vi "Set default values.vi"(8 "error in (no error)":errorcluster, 11 "device data model in":refnum<class "WebSocket Data Model.lvclass">) -> (0 "error out":errorcluster, 3 "device data model out":refnum<class "WebSocket Data Model.lvclass">)   [LabVIEW 2021, in "WebSockets.lvlib" / "WebSocket Data Model.lvclass"]
doc: "This VI ensures that the data model has at least 65,535 values of every type. This is required for certain modbus function codes."
uses:
  WebSocket Data Model.lvclass
  WebSocket Data Model.lvclass/WebSocket Data Model.ctl
  Type Definitions/Data Model.ctl
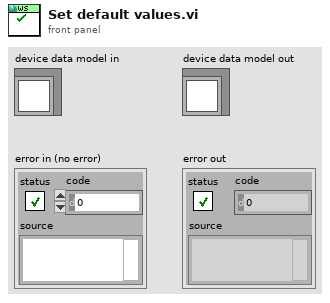
[diagram p1: front panel]
types:
  T1 = typedef "WebSockets.lvlib/WebSocket Data Model.lvclass/Data Model.ctl" = cluster{"UTC":u64, "Receive Binary Data":u8[], "Receive Text Data":string, "Send Binary Data":u8[], "Send Text Data":string, "ES":u8}
  T2 = typedef "Device Data Model.lvclass/N channel.ctl" = cluster{"N DI channel":i32, "N DO channel":i32, "N AI channel":i32, "N AO channel":i32}
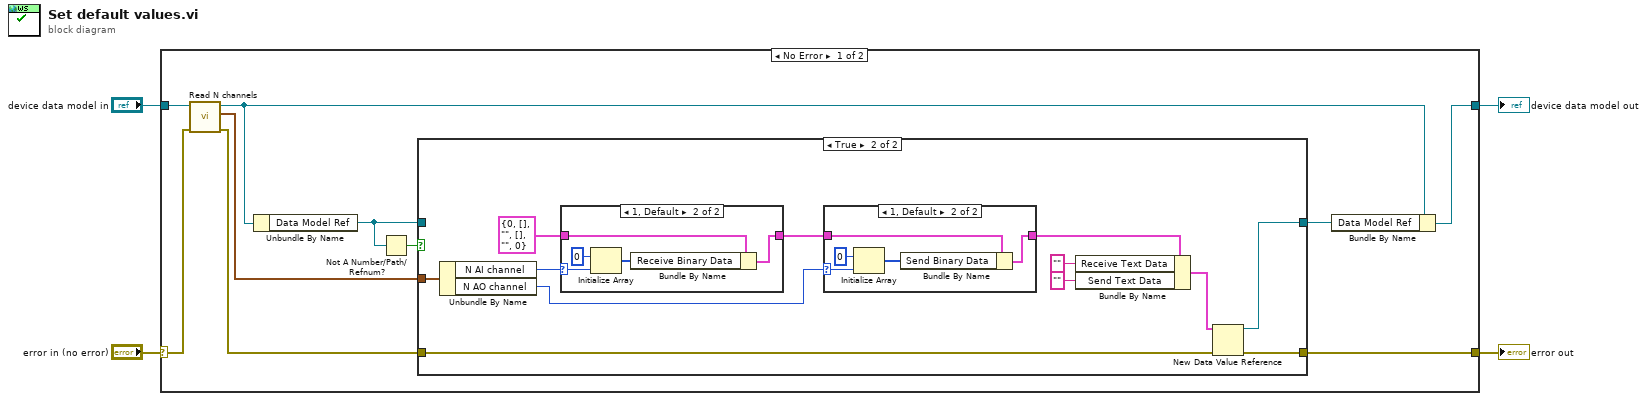
[diagram p0: block diagram]
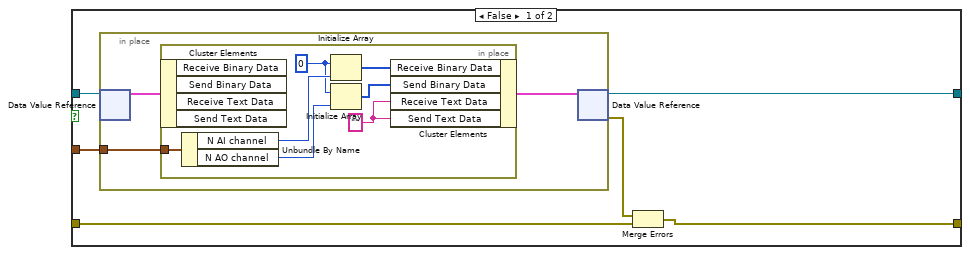
[diagram p2: hidden frame]
diagram:
  n1 = case shown="No Error" "error in (no error)" {
    selector: "error in (no error)" -> [w7 w56]
    tunnel: "device data model in" -> [w9 w55]
    tunnel: [w14 w55] -> w3
    tunnel: [w10 w56] -> w2
    frame No Error {
      n2 = call-dynamic "Read N channels.vi"("error in (no error)"=w7, "device data model in"=w9) -> ("error out"=w6:errorcluster, "N channel"=w5:T2, "device data model out"=w8:refnum<class "WebSocket Data Model.lvclass">)  [unwired: 7 in]
      n3 = Unbundle By Name(w8) -> ("Data Model Ref"=w12:refnum<data-value>)
      n4 = Not A Number/Path/Refnum?(number/path/refnum=w12) -> (NaN/Path/Refnum?=w11:bool)
      n5 = case shown="True" w11 {
        tunnel: w6 -> [w15 w42]
        tunnel: w12 -> [w20 _]
        tunnel: [w19 w40] -> w13
        tunnel: [w18 w41] -> w10
        tunnel: w5 -> [w16 w32]
        frame False {
          n6 = in-place {
            in-place-border: w16 -> [w22]
            n7 = in-place-dvr #1(w20) -> (w23:T1)  [unwired: 1 out]
            n8 = in-place {
              in-place-border: w22 -> [w30]
              w24 = "" ("Text Data")
              w26 = u8 0 ("Boolean")
              n9 = in-place-cluster #2(w23) -> ()  [unwired: 4 out]
              n10 = Unbundle By Name(w30) -> ("N AI channel"=w29:i32, "N AO channel"=w27:i32)
              n11 = Initialize Array(w26, w29) -> (w28:u8[])
              n12 = Initialize Array(w26, w27) -> (w25:u8[])
              n13 = in-place-cluster #2("Receive Binary Data"=w28, "Send Binary Data"=w25, "Receive Text Data"=w24, "Send Text Data"=w24) -> (w21:T1)
            }
            n14 = in-place-dvr #1(w21) -> (w19:refnum<data-value>, w17:errorcluster)
          }
          n15 = Merge Errors(w17, w15) -> (w18:errorcluster)
        }
        frame True {
          n16 = Unbundle By Name(w32) -> ("N AI channel"=w38:i32, "N AO channel"=w33:i32)
          n17 = case shown="1, Default" w38 {
            selector: w38 -> [_ w50]
            tunnel: T1 {"UTC"=0, "Receive Binary Data"=[], "Receive Text Data"="", "Send Binary Data"=[], "Send Text Data"="", "ES"=0} ("Data Model") -> [w49 w53]
            tunnel: [w49 w51] -> w35
            frame 0 {
            }
            frame 1, Default {
              n18 = Initialize Array(u8 0 ("Boolean"), w50) -> (w52:u8[])
              n19 = Bundle By Name(cluster=w53, "Receive Binary Data"=w52) -> (w51:T1)
            }
          }
          n20 = case shown="1, Default" w33 {
            selector: w33 -> [_ w44]
            tunnel: w35 -> [w43 w47]
            tunnel: [w43 w45] -> w34
            frame 0 {
            }
            frame 1, Default {
              n21 = Initialize Array(u8 0 ("Boolean"), w44) -> (w46:u8[])
              n22 = Bundle By Name(cluster=w47, "Send Binary Data"=w46) -> (w45:T1)
            }
          }
          n23 = Bundle By Name(cluster=w34, "Receive Text Data"="" ("Text Data"), "Send Text Data"="" ("Text Data")) -> (w31:T1)
          n24 = New Data Value Reference(data value=w31, error in=w42) -> (data value reference=w40:refnum<data-value>, error out=w41:errorcluster)
        }
      }
      n25 = Bundle By Name(cluster=w8, "Data Model Ref"=w13) -> (w14:refnum<class "WebSocket Data Model.lvclass">)
    }
    frame Error {
    }
  }
  "error out" <- w2
  "device data model out" <- w3
